vi "Interpolate 2D Scattered_Check Input 2D.vi"(10 "Yi":dbl[][](array[numeric]), 11 "Xi":dbl[][](array[numeric])) -> (0 "error":i32)   [LabVIEW 2020, in "NI_AAL_Interpolation.lvlib"]
uses:
  <vilib>/gmath/NI_AAL_Interpolation.lvlib
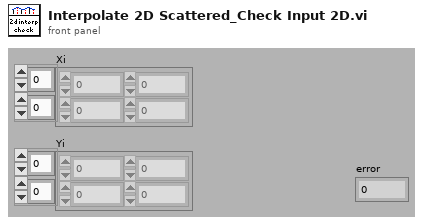
[diagram p1: front panel]
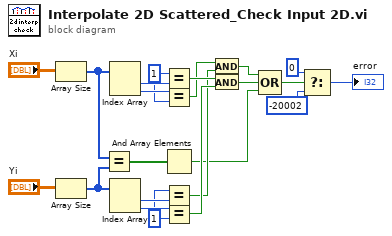
[diagram p0: block diagram]
diagram:
  w14 = 1 ("x")
  w17 = 1 ("x")
  n1 = Array Size(array="Xi") -> (size(s)=w4:i32[])
  n2 = Array Size(array="Yi") -> (size(s)=w10:i32[])
  n3 = Equal?(x=w4, y=w10) -> (x = y?=w20:bool[])
  n4 = Index Array(array=w4) -> (element #1=w19:i32, element #2=w18:i32)  [unwired: 2 in]
  n5 = Index Array(array=w10) -> (element #1=w16:i32, element #2=w15:i32)  [unwired: 2 in]
  n6 = Equal?(x=w17, y=w19) -> (x = y?=w13:bool)
  n7 = Equal?(x=w18, y=w17) -> (x = y?=w12:bool)
  n8 = And Array Elements(Boolean array=w20) -> (logical AND=w1:bool)
  n9 = Equal?(x=w14, y=w16) -> (x = y?=w8:bool)
  n10 = Equal?(x=w15, y=w14) -> (x = y?=w9:bool)
  n11 = And(x=w12, y=w8) -> (x .and. y?=w3:bool)
  n12 = And(x=w13, y=w9) -> (x .and. y?=w2:bool)
  n13 = Compound Arithmetic op=OR(w3, w2, w1) -> (w11:bool)
  n14 = Select(t=0, s=w11, f=-20002) -> (s? t:f=→"error":i32)
